vi "Initialize.vi"(8 "error in (no error)":errorcluster, 9 "Reset (True)":bool=TRUE, 10 "ID Query (True)":bool=TRUE, 11 "VISA resource name":refnum<visa-resource-name>) -> (0 "error out":errorcluster, 3 "VISA resource name out":refnum<visa-resource-name>)   [LabVIEW 2009, in "Agilent 8000 Series.lvlib"]
doc: "Establishes communication with the instrument and optionally performs an instrument identification query and/or an instrument reset. It also places the instrument in a default state needed for other instrument driver operations. Therefore, call this VI before calling other instrument driver VIs for this instrument. Generally, you need to call the Initialize VI only once at the beginning of an application."
uses:
  Agilent 8000 Series.lvlib
panel:
  # "(c) 2008 National Instruments.  ALL RIGHTS RESERVED."
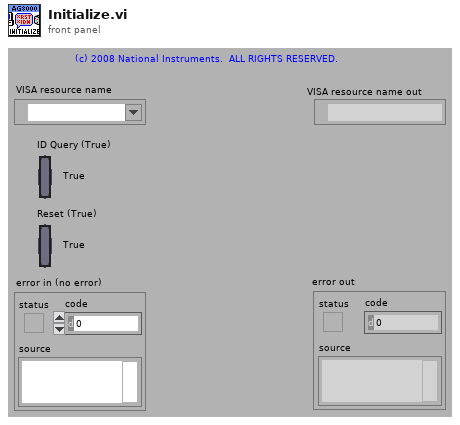
[diagram p1: front panel]
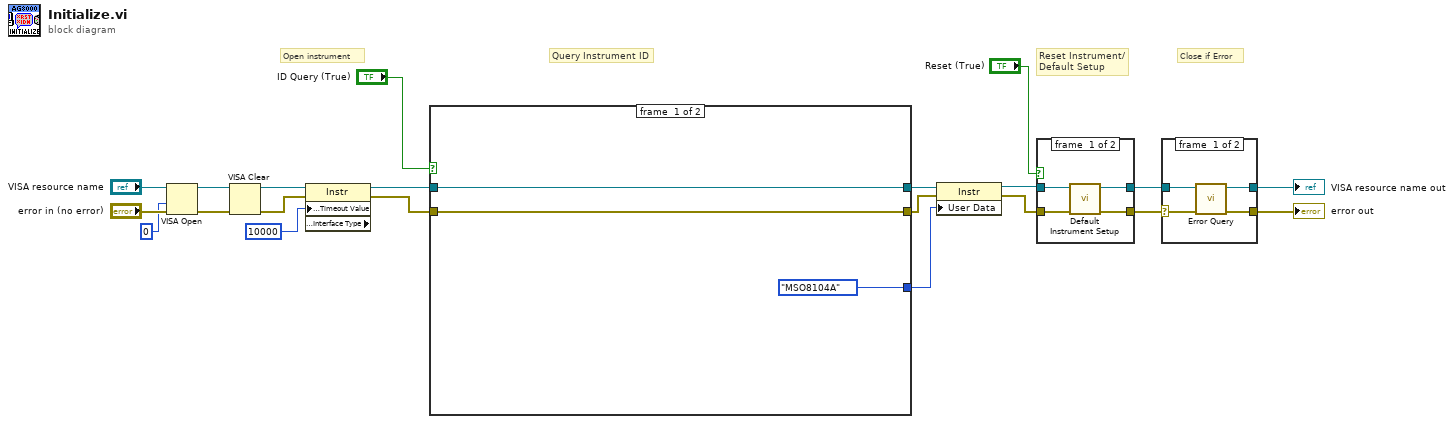
[diagram p0: block diagram]
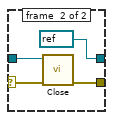
[diagram p2: hidden frame]
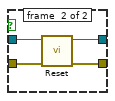
[diagram p3: hidden frame]
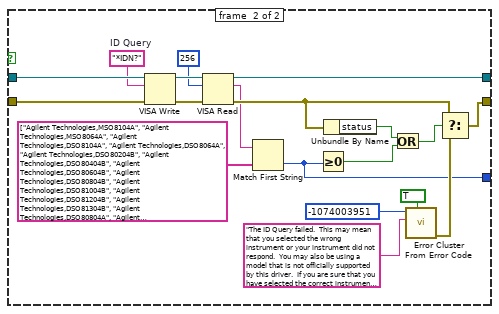
[diagram p4: hidden frame]
diagram:
  # "Close if Error"
  # "Query Instrument ID"
  # "Reset Instrument/\nDefault Setup"
  # "Open instrument"
  n1 = VISA Open(access mode=u32 0, error in (no error)="error in (no error)", VISA resource name="VISA resource name") -> (VISA resource name=w15:refnum<visa-resource-name>, error out=w14:errorcluster)  [unwired: 2 in]
  n2 = VISA Clear(VISA resource name=w15, error in (no error)=w14) -> (VISA resource name out=w13:refnum<visa-resource-name>, error out=w12:errorcluster)
  n3 = property class="Instr" props=["General Settings:Timeout Value", "Interface Information:Interface Type"](reference=w13, error in=w12, "General Settings:Timeout Value"=u32 10000) -> (reference out=w7:refnum<visa-resource-name>, error out=w6:errorcluster)  [unwired: 1 out]
  n4 = case shown="True" "ID Query (True)" {
    tunnel: [w23 w26] -> w5
    tunnel: [w24 w41] -> w4
    tunnel: w7 -> [w24 w42]
    tunnel: w6 -> [w23 w43]
    tunnel: [enum16{"MSO8104A"}."MSO8104A" w25] -> w1
    frame #0 {
    }
    frame #1 {
      w37 = "*IDN?"  # ID Query
      n5 = VISA Write(VISA resource name=w42, write buffer=w37, error in (no error)=w43) -> (VISA resource name out=w40:refnum<visa-resource-name>, error out=w39:errorcluster)  [unwired: 1 out]
      n6 = VISA Read(VISA resource name=w40, byte count=u32 256, error in (no error)=w39) -> (VISA resource name out=w41:refnum<visa-resource-name>, read buffer=w28:string, error out=w32:errorcluster)  [unwired: 1 out]
      n7 = Match First String(2:string[] ["Agilent Technologies,MSO8104A", "Agilent Technologies,MSO8064A", "Agilent Technologies,DSO8104A", "Agilent Technologies,DSO8064A", "Agilent Technologies,DSO80204B", "Agilent Technologies,DSO80404B", "Agilent Technologies,DSO80604B", "Agilent Technologies,DSO80804B", "Agilent Technologies,DSO81004B", "Agilent Technologies,DSO81204B", "Agilent Technologies,DSO81304B", "Agilent Technologies,DSO80804A", "Agilent Technologies,DSO81004A", "Agilent Technologies,DSO81204A", "Agilent Technologies,DSO81304A", "Agilent Technologies,DSO80304B"], 3:w28) -> (0:w25:i32)  [unwired: 1 out]
      n8 = Greater Or Equal To 0?(x=w25) -> (x >= 0?=w30:bool)
      n9 = Unbundle By Name(w32) -> ("status"=w31:bool)
      n10 = Or(x=w31, y=w30) -> (x .or. y?=w29:bool)
      n11 = call <vilib>:"Error Cluster From Error Code.vi"("show call chain? (False)"=TRUE, "error message (\"\")"="The ID Query failed.  This may mean that you selected the wrong instrument or your instrument did not respond.  You may also be using a model that is not officially supported by this driver.  If you are sure that you have selected the correct instrument and it is responding, try disabling the ID Query." ("Source (VI Name)"), "error code (0)"=-1074003951 ("Code")) -> ("error out"=w36:errorcluster)  [unwired: 6 in]
      n12 = Select(t=w32, s=w29, f=w36) -> (s? t:f=w26:errorcluster)
    }
  }
  n13 = property class="Instr"(reference=w4, error in=w5, "User Data"=w1) -> (reference out=w3:refnum<visa-resource-name>, error out=w2:errorcluster)
  n14 = case shown="True" "Reset (True)" {
    tunnel: w2 -> [w46 w48]
    tunnel: [w45 w51] -> w8
    tunnel: w3 -> [w47 w49]
    tunnel: [w44 w50] -> w9
    frame #0 {
      n15 = call "Default Instrument Setup.vi"("error in (no error)"=w46, "VISA resource name"=w47) -> ("error out"=w45:errorcluster, "VISA resource name out"=w44:refnum<visa-resource-name>)  [unwired: 8 in]
    }
    frame #1 {
      n16 = call "Reset.vi"("error in (no error)"=w48, "VISA resource name"=w49) -> ("error out"=w51:errorcluster, "VISA resource name out"=w50:refnum<visa-resource-name>)  [unwired: 8 in]
    }
  }
  n17 = case shown="Error" w8 {
    selector: w8 -> [w53 w57]
    tunnel: w9 -> [w52 w58]
    tunnel: [w55 refnum<visa-resource-name> refnum ("VISA resource name out")] -> w11
    tunnel: [w54 w59] -> w10
    frame #0 {
      n18 = call "Error Query.vi"("error in (no error)"=w53, "VISA resource name"=w52) -> ("error out"=w54:errorcluster, "VISA resource name out"=w55:refnum<visa-resource-name>)  [unwired: 6 in, 2 out]
    }
    frame #1 {
      n19 = call "Close.vi"("error in (no error)"=w57, "VISA resource name"=w58) -> ("error out"=w59:errorcluster)  [unwired: 9 in]
    }
  }
  "VISA resource name out" <- w11
  "error out" <- w10
